vi "Init Modal Dialogue GUI.vi"(4 "GUI Vertical Size (pixels)":i16=600, 6 "GUI Horizontal Size (pixels)":i16=800, 7 "Window Close (X) Button Enabled? (Default = True)":bool=TRUE, 8 "Error In":errorcluster, 9 "Background Colour (Default = 255,255,255)":u32(colorbox)=16777215, 10 "Window Title":string="Modal Dialogue", 11 "VI Refnum":refnum<vi>) -> (0 "Error Out":errorcluster)   [LabVIEW 2023, in "Error Manager.lvlib"]
doc: "This VI configures the Front Panel (the GUI) of the VI whose refnum is passed as an argument to the \"VI Refnum\" input (usually, the immediate caller VI)."
uses:
  Error Manager.lvlib
  <vilib>/Utility/miscctls.llb/LVPointTypeDef.ctl
  <vilib>/Utility/miscctls.llb/LVRectTypeDef.ctl
panel:
  # "Development\ncontrols/indicators useful for development and testing, but which are not outputs of the VI"
  # "Input\nInputs to the VI"
  # "Output\nOutputs of the VI"
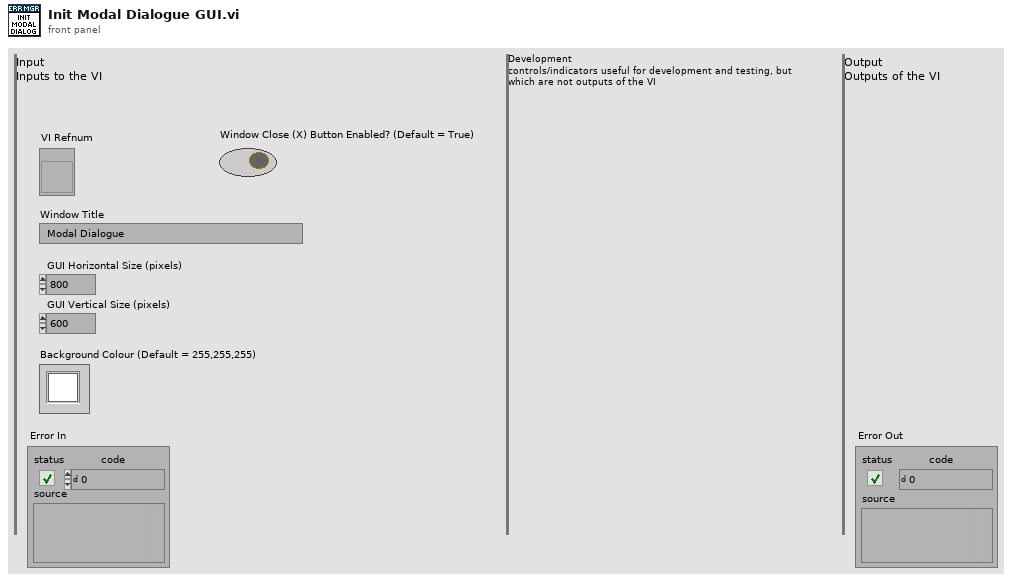
[diagram p1: front panel]
types:
  T1 = typedef "LVRectTypeDef.ctl" = cluster{"Left":i16, "Top":i16, "Right":i16, "Bottom":i16}
  T2 = typedef "LVPointTypeDef.ctl" = cluster{"Horizontal":i16, "Vertical":i16}
  T3 = enum32{"Invalid", "Default", "Floating", "Floating/Auto-Hide", "Modal"}
  T4 = enum32{"Invalid", "Standard", "Closed", "Hidden", "Minimized", "Maximized"}
  T5 = enum16{"Always On", "Always Off", "Off While Running"}
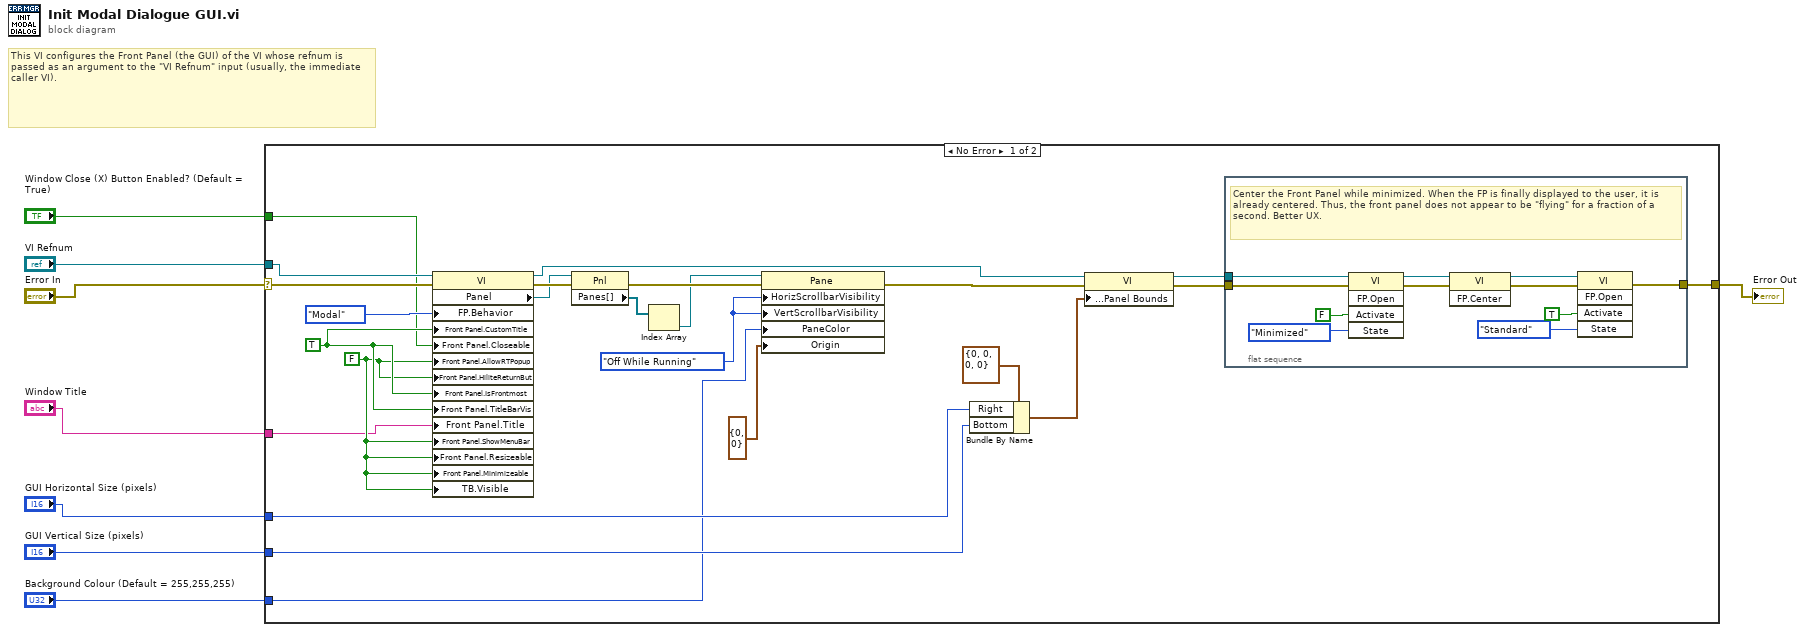
[diagram p0: block diagram]
diagram:
  # "This VI configures the Front Panel (the GUI) of the VI whose refnum is passed as an argument to the \"VI Refnum\" input (usually, the immediate caller VI)."
  n1 = case shown="No Error" "Error In" {
    selector: "Error In" -> [w32 w44]
    tunnel: [w21 w44] -> w7
    tunnel: "VI Refnum" -> [w30 _]
    tunnel: "Window Title" -> [w13 _]
    tunnel: "GUI Horizontal Size (pixels)" -> [w12 _]
    tunnel: "GUI Vertical Size (pixels)" -> [w11 _]
    tunnel: "Window Close (X) Button Enabled? (Default = True)" -> [w10 _]
    tunnel: "Background Colour (Default = 255,255,255)" -> [w9 _]
    frame No Error {
      w23 = T5."Off While Running" ("Horizontal Scrollbar Visibility")
      w22 = FALSE
      w28 = TRUE
      n2 = property class="VI"(reference=w30, error in=w32, "FP.Behavior"=T3."Modal" ("Front Panel Window:Behavior"), "Front Panel.CustomTitle"=w28, "Front Panel.Closeable"=w10, "Front Panel.AllowRTPopup"=w22, "Front Panel.HiliteReturnBut"=w22, "Front Panel.IsFrontmost"=w28, "Front Panel.TitleBarVis"=w28, "Front Panel.Title"=w13, "Front Panel.ShowMenuBar"=w22, "Front Panel.Resizeable"=w22, "Front Panel.Minimizeable"=w22, "TB.Visible"=w22) -> (reference out=w17:refnum<vi>, error out=w31:errorcluster, "Panel"=w26:refnum<vi>)
      n3 = property class="Pnl"(reference=w26, error in=w31) -> (error out=w27:errorcluster, "Panes[]"=w25:refnum<vi>[])  [unwired: 1 out]
      n4 = Index Array(array=w25) -> (element=w24:refnum<vi>)  [unwired: 1 in]
      n5 = property class="Pane"(reference=w24, error in=w27, "HorizScrollbarVisibility"=w23, "VertScrollbarVisibility"=w23, "PaneColor"=w9, "Origin"=T2 {"Horizontal"=0, "Vertical"=0}) -> (error out=w19:errorcluster)  [unwired: 1 out]
      n6 = Bundle By Name(cluster=T1 {"Left"=0, "Top"=0, "Right"=0, "Bottom"=0} ("Front Panel Window:Panel Bounds"), "Right"=w12, "Bottom"=w11) -> (w15:T1)
      n7 = property on="Property Node" class="VI"(reference=w17, error in=w19, "Front Panel Window:Panel Bounds"=w15) -> (reference out=w14:refnum<vi>, error out=w18:errorcluster)
      n8 = flat-sequence {
        tunnel: [w43] -> w21
        tunnel: w18 -> [w40]
        tunnel: w14 -> [w36]
        frame #0 {
          # "Center the Front Panel while minimized. When the FP is finally displayed to the user, it is already centered. Thus, the front panel does not appear to be \"flying\" for a fraction of a second. Better UX."
          n9 = invoke class="VI" method="FP.Open"(reference=w36, error in=w40, "Activate"=FALSE ("Activate?"), "State"=T4."Minimized") -> (reference out=w35:refnum<vi>, error out=w37:errorcluster)  [unwired: 1 in, 3 out]
          n10 = invoke class="VI" method="FP.Center"(reference=w35, error in=w37) -> (reference out=w38:refnum<vi>, error out=w39:errorcluster)  [unwired: 1 in, 1 out]
          n11 = invoke class="VI" method="FP.Open"(reference=w38, error in=w39, "Activate"=TRUE ("Activate?"), "State"=T4."Standard") -> (error out=w43:errorcluster)  [unwired: 1 in, 4 out]
        }
      }
    }
    frame Error {
    }
  }
  "Error Out" <- w7
